vi "NS_SetProperty.vi"(0 "object in":refnum<class "NativeSubTemplate.lvclass">, 1 "Property":bool, 5 "error in (no error)":errorcluster) -> (14 "object out":refnum<class "NativeSubTemplate.lvclass">, 19 "error out":errorcluster)   [LabVIEW 2020, in "NativeSubTemplate.lvclass"]
uses:
  <resource>/Framework/Providers/Open_GDS/ClassProviders/Provider_LvNativeClass/Templates/NativeSubTemplate/NativeSubTemplate.lvclass
  <resource>/Framework/Providers/Open_GDS/ClassProviders/Provider_LvNativeClass/Templates/NativeSubTemplate/NativeSubTemplate.lvclass/NativeSubTemplate.ctl
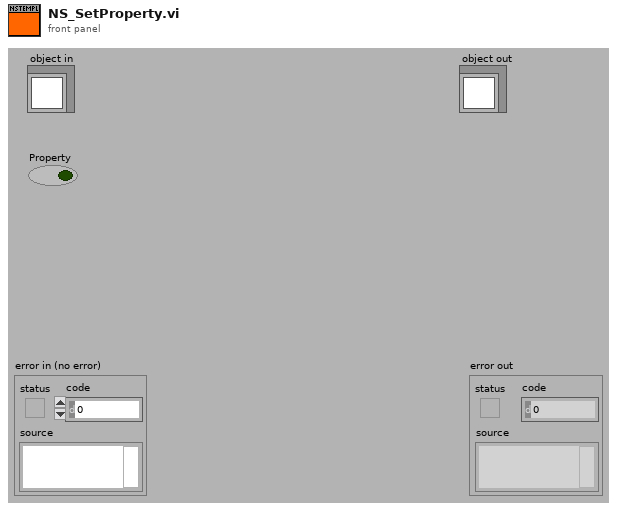
[diagram p1: front panel]
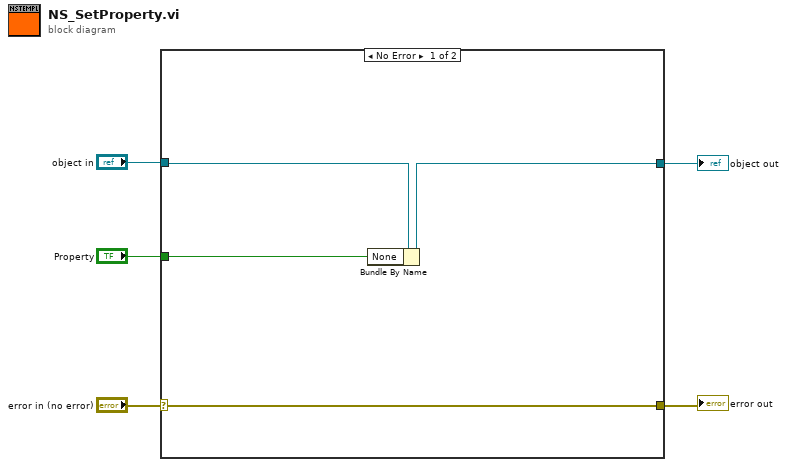
[diagram p0: block diagram]
diagram:
  n1 = case shown="No Error" "error in (no error)" {
    selector: "error in (no error)" -> [w8 w11]
    tunnel: [w8 w11] -> w4
    tunnel: [w6 w10] -> w2
    tunnel: "object in" -> [w7 w10]
    tunnel: "Property" -> [w9 _]
    frame No Error {
      n2 = Bundle By Name(cluster=w7, "None"=w9) -> (w6:refnum<class "NativeSubTemplate.lvclass">)
    }
    frame Error {
    }
  }
  "error out" <- w4
  "object out" <- w2
